vi "CRYCheck HT Option.vi"(9 "Option Array In":bool[](array[boolean]), 10 "Type":u16, 11 "Algorithm":u16) -> (3 "Option Array Out":bool[](array[boolean]))   [LabVIEW 2013]
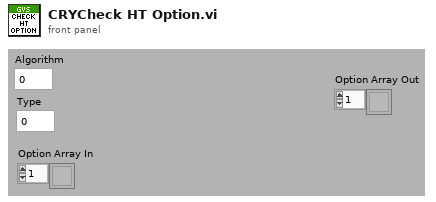
[diagram p1: front panel]
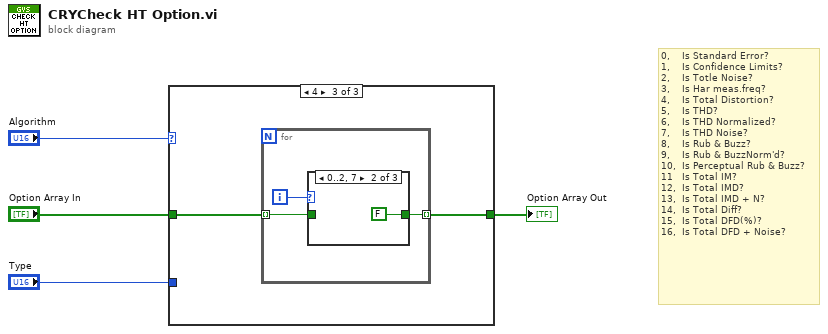
[diagram p0: block diagram]
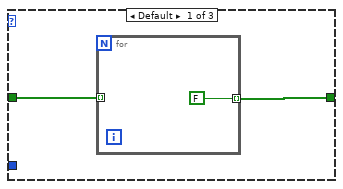
[diagram p2: hidden frame]
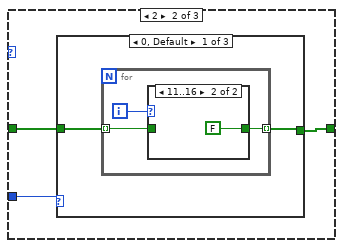
[diagram p3: hidden frame]
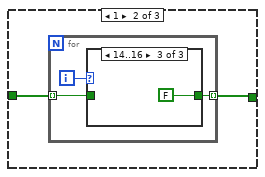
[diagram p5: hidden frame]
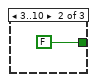
[diagram p7: hidden frame]
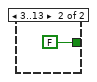
[diagram p9: hidden frame]
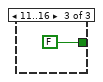
[diagram p11: hidden frame]
diagram:
  # "0,    Is Standard Error?\n1,    Is Confidence Limits?\n2,    Is Totle Noise?\n3,    Is Har meas.freq?\n4,    Is Total Distortion?\n5,    Is THD?\n6,    Is THD Normalized?\n7,    Is THD Noise?\n8,    Is Rub & Buzz?\n9,    Is Rub & BuzzNorm'd?\n10,  Is Perceptual Rub & Buzz?\n11   Is Total IM?\n12,  Is Total IMD?\n13,  Is Total IMD + N?\n14,  Is Total Diff?\n15,  Is Total DFD(%)?\n16,  Is Total DFD + Noise?"
  n1 = case shown="4" "Algorithm" {
    tunnel: "Option Array In" -> [w6 w10 w34]
    tunnel: "Type" -> [_ w9 _]
    tunnel: [w5 w8 w33] -> w1
    frame Default {
      n2 = for {
        tunnel: w6 -> [_] mode=indexing
        tunnel: [FALSE ("Is Har meas.freq? 2")] -> w5 mode=indexing
      }
    }
    frame 2 {
      n3 = case shown="0, Default" w9 {
        tunnel: w10 -> [w12 w19 w27]
        tunnel: [w11 w18 w26] -> w8
        frame 0, Default {
          n4 = for {
            tunnel: w12 -> [w14] mode=indexing
            tunnel: [w13] -> w11 mode=indexing
            i -> [w15]
            n5 = case shown="11..16" w15 {
              tunnel: w14 -> [w16 _]
              tunnel: [w16 FALSE ("Is Har meas.freq? 2")] -> w13
              frame Default {
              }
              frame 11..16 {
              }
            }
          }
        }
        frame 1 {
          n6 = for {
            tunnel: w19 -> [w21] mode=indexing
            tunnel: [w20] -> w18 mode=indexing
            i -> [w22]
            n7 = case shown="14..16" w22 {
              tunnel: w21 -> [w23 _ _]
              tunnel: [w23 FALSE ("Is Har meas.freq? 2") FALSE ("Is Har meas.freq? 2")] -> w20
              frame Default {
              }
              frame 3..10 {
              }
              frame 14..16 {
              }
            }
          }
        }
        frame 2 {
          n8 = for {
            tunnel: w27 -> [w29] mode=indexing
            tunnel: [w28] -> w26 mode=indexing
            i -> [w30]
            n9 = case shown="Default" w30 {
              tunnel: w29 -> [w31 _]
              tunnel: [w31 FALSE ("Is Har meas.freq? 2")] -> w28
              frame Default {
              }
              frame 3..13 {
              }
            }
          }
        }
      }
    }
    frame 4 {
      n10 = for {
        tunnel: w34 -> [w36] mode=indexing
        tunnel: [w35] -> w33 mode=indexing
        i -> [w37]
        n11 = case shown="0..2, 7" w37 {
          tunnel: w36 -> [w38 _ _]
          tunnel: [w38 FALSE ("Is Har meas.freq? 2") FALSE ("Is Har meas.freq? 2")] -> w35
          frame Default {
          }
          frame 0..2, 7 {
          }
          frame 11..16 {
          }
        }
      }
    }
  }
  "Option Array Out" <- w1
